vi "Read_param.vi"() -> ()   [LabVIEW 2018]
uses:
  Init/AllPath.vi
  <vilib>/Utility/file.llb/Read Delimited Spreadsheet (string).vi
panel:
  out "数组":string[](array[string])
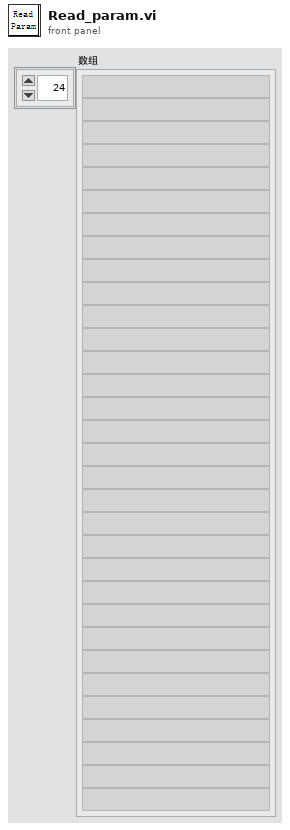
[diagram p1: front panel]
types:
  T1 = cluster{"能量/功率":path, " 示波器":path, " 光谱仪":path, "偏振":path, "近远场":cluster{" 近场图片":path, " 远场图片":path, "发散角数据":path}, "参数":path, " 基路径":path, "文件名信息":path, "输出模板路径":path, "输出报告路径":path, "位置信息路径":path}
  T2 = typedef "IMAQ Image.ctl" = refnum<image>
  T3 = cluster{"示波器":cluster{"Channel (0:Channel 1)":enum16{"Channel 1", "Channel 2", "Channel 3", "Channel 4"}, "电压范围":dbl, "触发电压":dbl, "时间范围":dbl, " 示波器VISA":refnum<visa-resource-name>, "时间范围 标签":u64, "电压范围 标签":u64, "触发电压 标签":u64, "输入阻抗/Ω":u64, "示波器类型":bool}, "光谱仪":cluster{"SpecDataReference":refnum<queue>, "grating center":dbl, "Exposure Time (s)":dbl, "是否进行详细设置":bool, " 开始通信检查":bool, "通信成功？":bool, "波长":dbl, "LightField Automation out":refnum<class "LightField Automation.lvclass">}, " 近场相机":cluster{"曝光时间/us":dbl, "IP 地址":string, "ImageData":T2, " 曝光最大":i32, " 曝光最小":i32, "Camera Source":refnum<k21>, "近场X范围1":dbl, "近场Y范围1":dbl, "单个像元大小/um":dbl, "相机距离原点位置":dbl[], "是否测量发散角":bool, "光束类型(发散T)":bool, "聚焦透镜焦距mm":dbl, "近场X范围2":dbl, "近场Y范围2":dbl}, " 偏振仪":cluster{"电压范围":u64, "触发电压":u64, "时间范围":u64, "波长范围":enum16{"可见光 400-700nm", "近红外 700-1100nm"}, "可见光偏振测量仪VISA":refnum<visa-resource-name>, "近红外偏振测量仪VISA":refnum<visa-resource-name>}, " 功率计":cluster{"通道":enum16{"Channel 1", "Channel 2"}, "工作波长":u32, "单位":u64, "时间范围":u64, "IP地址":string, "端口":u32, "是否需要散射片":bool}, "能量计":cluster{"通道":enum16{"Channel 1", "Channel 2"}, "工作波长":u32, "单位":u64, "时间范围":u64, "IP地址":string, "端口":u32, "能量计量程":enum16{"200uJ", "20uJ", "2uJ", "200nJ"}}, "电机":cluster{"Channel (0:Channel 1)":enum16{"Channel 1", "Channel 2", "Channel 3", "Channel 4"}, "电压范围":u64, "触发电压":u64, "时间范围":u64}, " 远场相机":cluster{"曝光时间/us":i32, "IP 地址":string, "ImageData":T2, "  增益最大":i32, "  增益最小":i32, " 曝光最大":i32, " 曝光最小":i32, "ImageData B":T2, "是否远场测量":bool}}
  T4 = typedef "衰减片电机位置枚举器.ctl" = enum16{"0倍", "10倍", "100倍", "1000倍"}
  T5 = cluster{"激光器型号":string, "X":dbl, "Y":dbl, "Z":dbl, "Rotate":dbl, "Pitching":dbl, "DivergeAngle":dbl, "衰减片位置":cluster{"小积分球位置":T4, "偏振仪位置 ":T4, "近场相机位置 ":T4, "远场相机位置":T4}, "Type":string, "Serial":string}
  T6 = cluster{"Selected Index []":i32[], "Selected Items":string[], " 所有任务":string[], "任务布尔":bool[]}
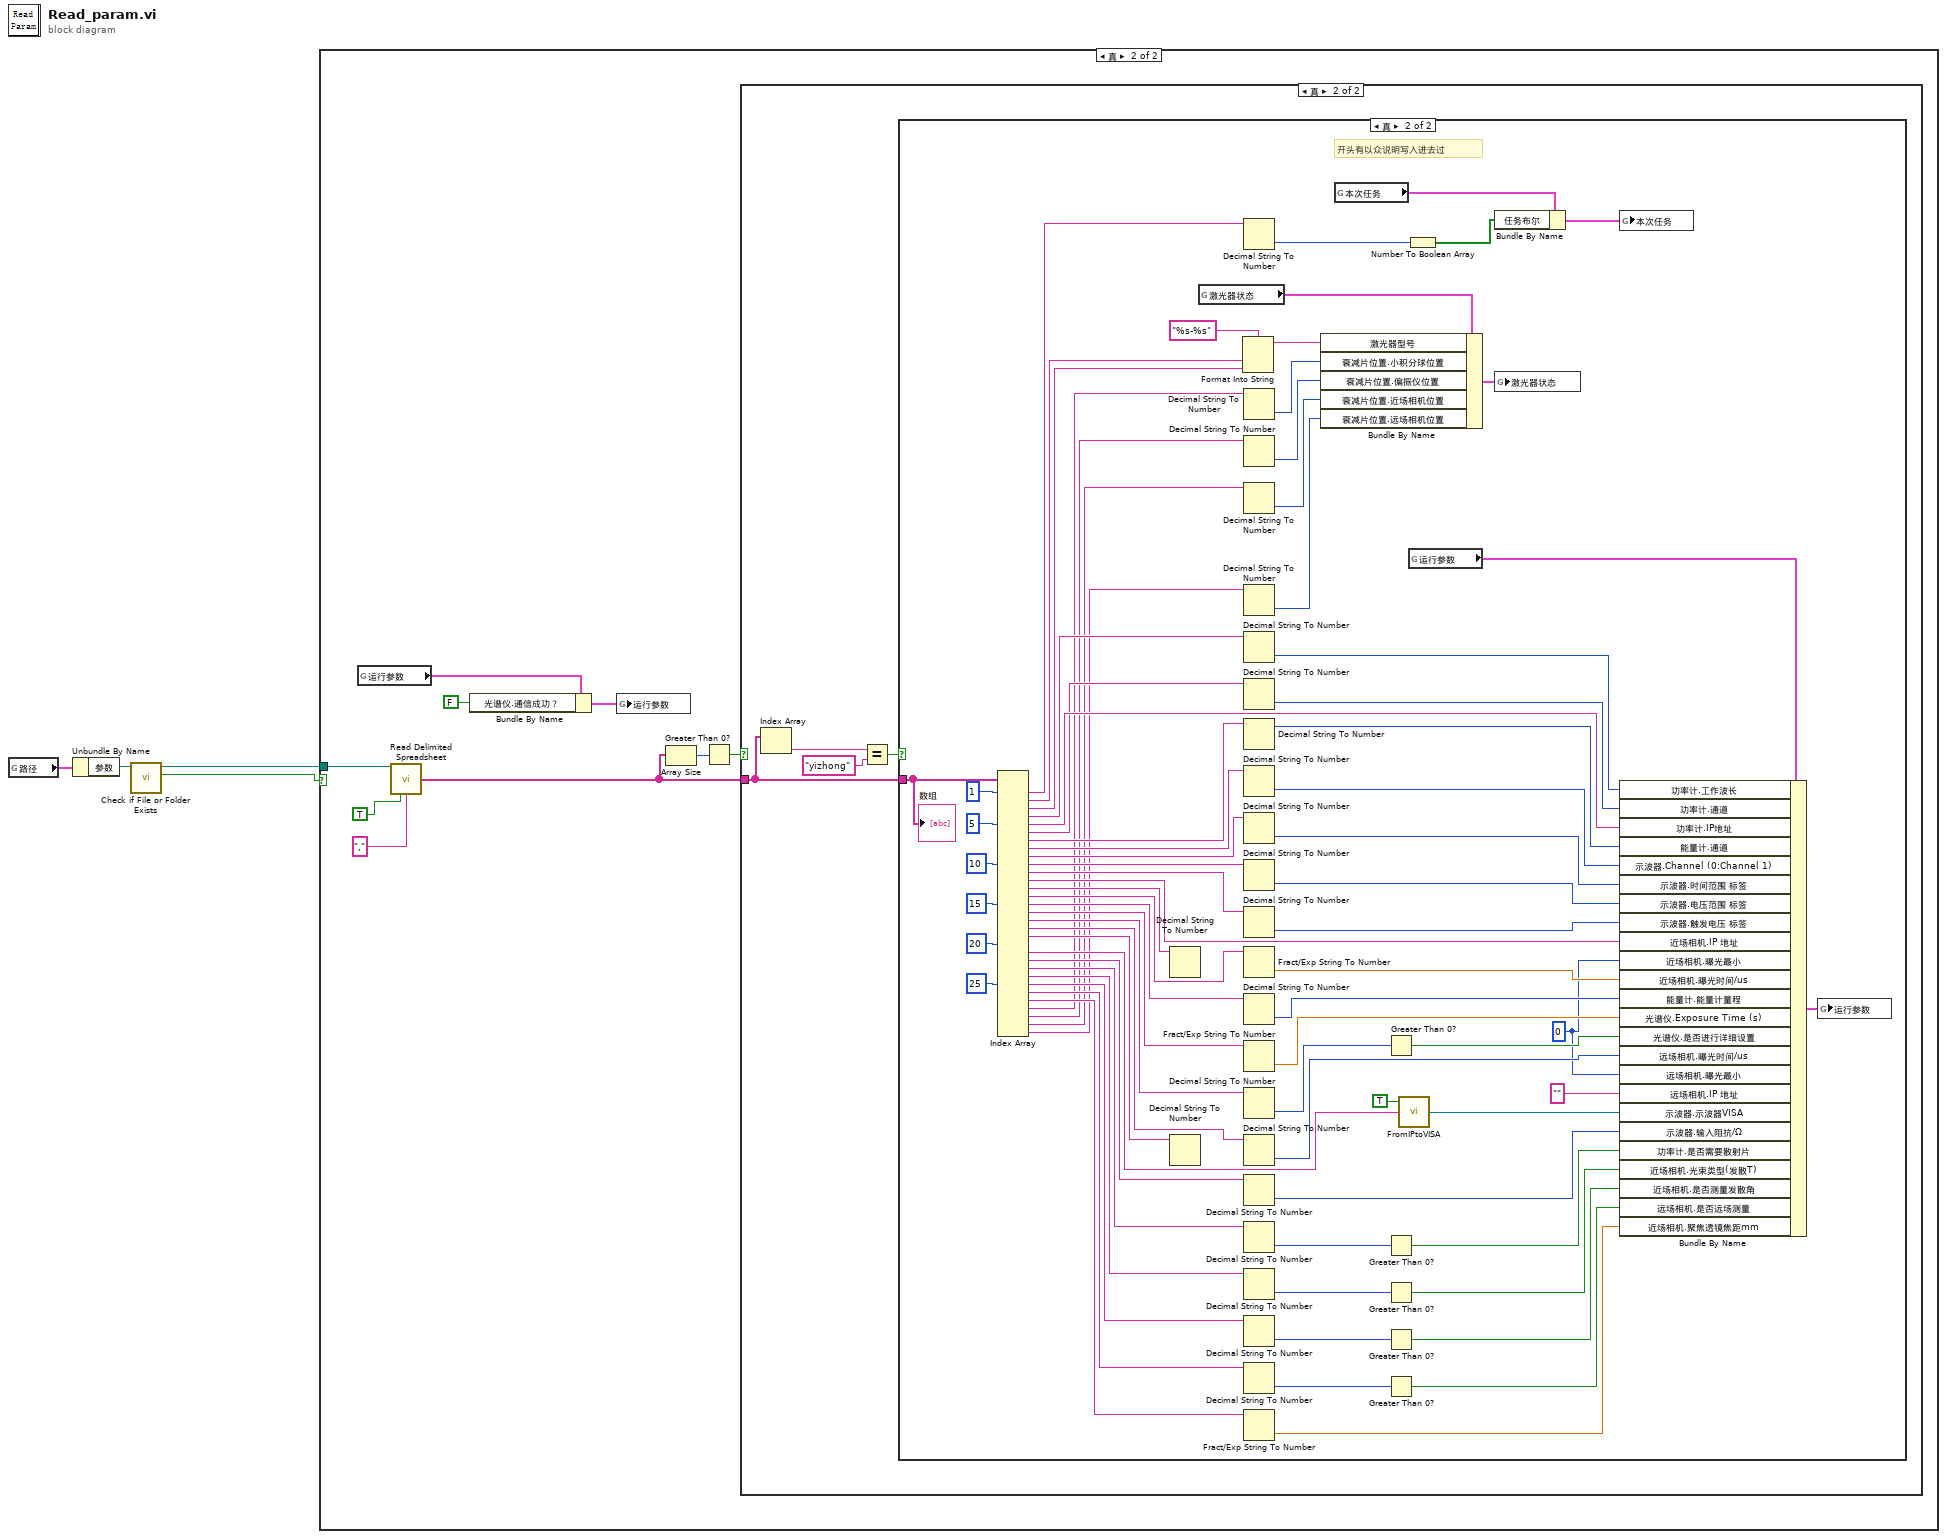
[diagram p0: block diagram]
diagram:
  n1 = global read "AllPath.vi" "路径"() -> (w4:T1)
  n2 = Unbundle By Name(w4) -> ("参数"=w3:path)
  n3 = call <vilib>:"Check if File or Folder Exists.vi"("path"=w3) -> ("file or folder exists?"=w1:bool, "dup path"=w2:path)  [unwired: 8 in, 1 out]
  n4 = case shown="真" w1 {
    tunnel: w2 -> [_ w9]
    frame False {
    }
    frame True {
      n5 = global read "参数.vi" "运行参数"() -> (w8:T3)
      n6 = call-poly <vilib>:"Read Delimited Spreadsheet.vi"("file path (dialog if empty)"=w9, "transpose? (F)"=TRUE, "delimiter (\\t)"="," ("delimiter (\\t)")) -> ("first row"=w13:string[])  [unwired: 7 in, 5 out]
      n7 = Bundle By Name(cluster=w8, "光谱仪.通信成功？"=FALSE ("光谱仪.通信检查完毕")) -> (w6:T3)
      n8 = global write "参数.vi" "运行参数"(w6) -> ()
      n9 = Array Size(array=w13) -> (size(s)=w12:i32)
      n10 = Greater Than 0?(x=w12) -> (x > 0?=w11:bool)
      n11 = case shown="真" w11 {
        tunnel: w13 -> [_ w17]
        frame False {
        }
        frame True {
          n12 = Index Array(array=w17) -> (element=w16:string)  [unwired: 1 in]
          n13 = Equal?(x=w16, y="yizhong" ("元素")) -> (x = y?=w14:bool)
          n14 = case shown="真" w14 {
            tunnel: w17 -> [_ w31]
            frame False {
            }
            frame True {
              w34 = 0 ("近场相机. 曝光最大")
              # "开头有以众说明写入进去过"
              n15 = Index Array(array=w31, index #1=1 ("索引"), index #5=5 ("索引"), index #10=10 ("索引"), index #15=15 ("索引"), index #20=20 ("索引"), index #25=25 ("索引")) -> (element #1=w70:string, element #2=w73:string, element #3=w72:string, element #4=w93:string, element #5=w65:string, element #6=w64:string, element #7=w90:string, element #8=w88:string, element #9=w86:string, element #10=w85:string, element #11=w84:string, element #12=w79:string, element #13=w80:string, element #14=w33:string, element #15=w63:string, element #16=w61:string, element #17=w60:string, element #18=w56:string, element #19=w55:string, element #21=w52:string, element #22=w50:string, element #23=w47:string, element #24=w25:string, element #25=w24:string, element #26=w23:string, element #27=w22:string, element #28=w21:string, element #29=w20:string, element #30=w19:string, element #31=w18:string)  [unwired: 25 in, 1 out]
              n16 = Decimal String To Number(string=w80) -> ()  [unwired: 2 in, 2 out]
              n17 = Decimal String To Number(string=w55) -> ()  [unwired: 2 in, 2 out]
              n18 = global read "参数.vi" "激光器状态"() -> (w95:T5)
              n19 = Format Into String(format string="%s-%s" ("格式字符串"), w73, w72) -> (resulting string=w75:string)  [unwired: 2 in, 1 out]
              n20 = Decimal String To Number(string=w70) -> (number=w69:i32)  [unwired: 2 in, 1 out]
              n21 = Decimal String To Number(string=w21) -> (number=w38:i32)  [unwired: 2 in, 1 out]
              n22 = Decimal String To Number(string=w20) -> (number=w37:i32)  [unwired: 2 in, 1 out]
              n23 = Decimal String To Number(string=w19) -> (number=w36:i32)  [unwired: 2 in, 1 out]
              n24 = Decimal String To Number(string=w18) -> (number=w35:i32)  [unwired: 2 in, 1 out]
              n25 = Decimal String To Number(string=w93) -> (number=w92:i32)  [unwired: 2 in, 1 out]
              n26 = Decimal String To Number(string=w64) -> (number=w91:i32)  [unwired: 2 in, 1 out]
              n27 = Decimal String To Number(string=w90) -> (offset past number=w89:i32)  [unwired: 2 in, 1 out]
              n28 = Decimal String To Number(string=w88) -> (number=w87:i32)  [unwired: 2 in, 1 out]
              n29 = Decimal String To Number(string=w86) -> (number=w83:i32)  [unwired: 2 in, 1 out]
              n30 = Decimal String To Number(string=w85) -> (number=w82:i32)  [unwired: 2 in, 1 out]
              n31 = Decimal String To Number(string=w84) -> (number=w81:i32)  [unwired: 2 in, 1 out]
              n32 = Fract/Exp String To Number(string=w33) -> (number=w78:dbl)  [unwired: 3 in, 1 out]
              n33 = Decimal String To Number(string=w63) -> (number=w62:i32)  [unwired: 2 in, 1 out]
              n34 = Fract/Exp String To Number(string=w61) -> (number=w59:dbl)  [unwired: 3 in, 1 out]
              n35 = Decimal String To Number(string=w60) -> (number=w58:i32)  [unwired: 2 in, 1 out]
              n36 = Decimal String To Number(string=w56) -> (number=w54:i32)  [unwired: 2 in, 1 out]
              n37 = Decimal String To Number(string=w50) -> (number=w49:i32)  [unwired: 2 in, 1 out]
              n38 = Decimal String To Number(string=w47) -> (number=w48:i32)  [unwired: 2 in, 1 out]
              n39 = Decimal String To Number(string=w25) -> (number=w45:i32)  [unwired: 2 in, 1 out]
              n40 = Decimal String To Number(string=w24) -> (number=w43:i32)  [unwired: 2 in, 1 out]
              n41 = Decimal String To Number(string=w23) -> (number=w41:i32)  [unwired: 2 in, 1 out]
              n42 = Fract/Exp String To Number(string=w22) -> (number=w39:dbl)  [unwired: 3 in, 1 out]
              n43 = Bundle By Name(cluster=w95, "激光器型号"=w75, "衰减片位置.小积分球位置"=w38, "衰减片位置.偏振仪位置"=w37, "衰减片位置.近场相机位置"=w36, "衰减片位置.远场相机位置"=w35) -> (w76:T5)
              n44 = global read "参数.vi" "本次任务"() -> (w68:T6)
              n45 = Greater Than 0?(x=w58) -> (x > 0?=w57:bool)
              n46 = Greater Than 0?(x=w48) -> (x > 0?=w46:bool)
              n47 = Greater Than 0?(x=w45) -> (x > 0?=w44:bool)
              n48 = Greater Than 0?(x=w43) -> (x > 0?=w42:bool)
              n49 = Greater Than 0?(x=w41) -> (x > 0?=w40:bool)
              n50 = call "FromIPtoVISA.vi"("IP input"=w52, "IP to VISA?"=TRUE) -> ("VISA out"=w51:refnum<visa-resource-name>)  [unwired: 2 in, 1 out]
              n51 = Number To Boolean Array(number=w69) -> (Boolean array=w67:bool[])
              n52 = global read "参数.vi" "运行参数"() -> (w94:T3)
              n53 = Bundle By Name(cluster=w68, "任务布尔"=w67) -> (w66:T6)
              n54 = global write "参数.vi" "激光器状态"(w76) -> ()
              n55 = global write "参数.vi" "本次任务"(w66) -> ()
              n56 = Bundle By Name(cluster=w94, "功率计.工作波长"=w92, "功率计.通道"=w91, "功率计.IP地址"=w65, "能量计.通道"=w89, "示波器.Channel (0:Channel 1)"=w87, "示波器.时间范围 标签"=w83, "示波器.电压范围 标签"=w82, "示波器.触发电压 标签"=w81, "近场相机.IP 地址"=w79, "近场相机.曝光最小"=w34, "近场相机.曝光时间/us"=w78, "能量计.能量计量程"=w62, "光谱仪.Exposure Time (s)"=w59, "光谱仪.是否进行详细设置"=w57, "远场相机.曝光时间/us"=w54, "远场相机.曝光最小"=w34, "远场相机.IP 地址"="", "示波器.示波器VISA"=w51, "示波器.输入阻抗/Ω"=w49, "功率计.是否需要散射片"=w46, "近场相机.光束类型(发散T)"=w44, "近场相机.是否测量发散角"=w42, "远场相机.是否远场测量"=w40, "近场相机.聚焦透镜焦距mm"=w39) -> (w77:T3)
              n57 = global write "参数.vi" "运行参数"(w77) -> ()
              "数组" <- w31
            }
          }
        }
      }
    }
  }
